vi "niDAQmx Get Channel Property.vi"   [LabVIEW 2021, in "Session Management niDAQmx.lvlib" / "Session Factory.lvclass"]
doc: "Property node to get information from NI-DAQmx channels."
uses:
  Session Factory.lvclass
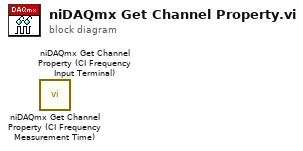
[diagram p0: block diagram]
diagram:
  n1 = call "niDAQmx Get Channel Property (CI Frequency Measurement Time).vi"() -> ()  [unwired: 13 in, 3 out]
  n2 = call "niDAQmx Get Channel Property (CI Frequency Input Terminal).vi"() -> ()  [unwired: 13 in, 3 out]
